vi "DSF.Engine.Transfer Group.Set ID.vi"(10 "id":i32, 11 "Transfer Group in":refnum<class "DSF.Engine.Transfer Group.lvclass">) -> (3 "Transfer Group out":refnum<class "DSF.Engine.Transfer Group.lvclass">)   [LabVIEW 2017, in "DSF.Engine.lvlib" / "DSF.Engine.Transfer Group.lvclass"]
uses:
  DSF.Engine.Transfer Group.lvclass
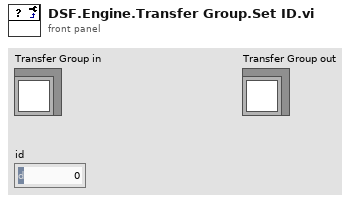
[diagram p1: front panel]
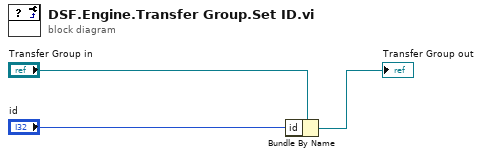
[diagram p0: block diagram]
diagram:
  n1 = Bundle By Name(cluster="Transfer Group in", "id"="id") -> (→"Transfer Group out":refnum<class "DSF.Engine.Transfer Group.lvclass">)
